vi "Cache Directive String.vi"(10 "Cache Directive":T1=enum."None (no-store)") -> (2 "Cache-Control Directive":string[](array[string]), 5 "no-store?":bool)   [LabVIEW 2020, in "HTTP Utils.lvlib"]
uses:
  HTTP Utils.lvlib
  Cache Directive.ctl
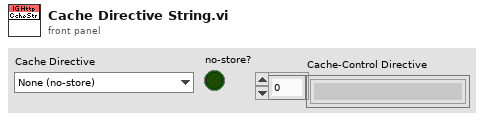
[diagram p1: front panel]
types:
  T1 = typedef "HTTP Utils.lvlib/Cache Directive.ctl" = enum16{"Not Specified", "None (no-store)", "Always Validate (no-cache)", "Private Only (private)", "Always Allow (public)"}
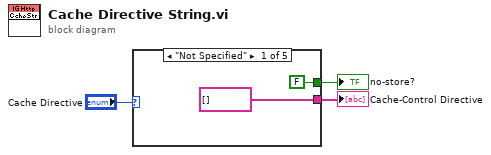
[diagram p0: block diagram]
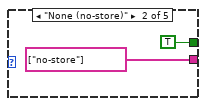
[diagram p2: hidden frame]
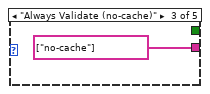
[diagram p3: hidden frame]
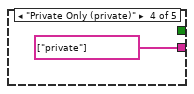
[diagram p4: hidden frame]
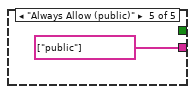
[diagram p5: hidden frame]
diagram:
  n1 = case shown="\"Not Specified\"" "Cache Directive" {
    tunnel: [string[] [] string[] ["no-store"] string[] ["no-cache"] string[] ["private"] string[] ["public"]] -> w2
    tunnel: [FALSE TRUE _ _ _] -> w1
    frame "Not Specified" {
    }
    frame "None (no-store)" {
    }
    frame "Always Validate (no-cache)" {
    }
    frame "Private Only (private)" {
    }
    frame "Always Allow (public)" {
    }
  }
  "Cache-Control Directive" <- w2
  "no-store?" <- w1
